vi "BlockInput8-2.vi"(3 "error in (no error)":errorcluster, 5 "BlockInput?":bool=TRUE) -> (0 "error in (no error) 2":errorcluster)   [LabVIEW 2014]
uses:
  user32.dll
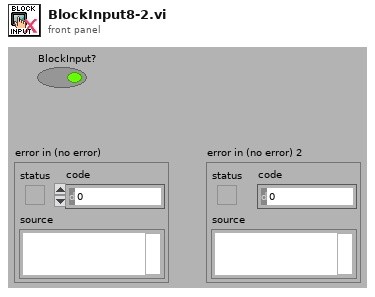
[diagram p1: front panel]
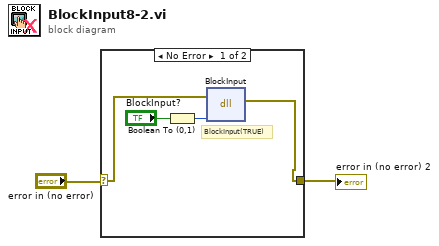
[diagram p0: block diagram]
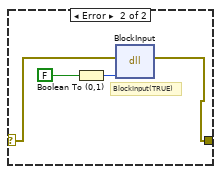
[diagram p2: hidden frame]
diagram:
  n1 = case shown="No Error" "error in (no error)" {
    selector: "error in (no error)" -> [w3 w8]
    tunnel: [w4 w7] -> w1
    frame No Error {
      # "BlockInput(TRUE)"
      n2 = Boolean To (0,1)(Boolean="BlockInput?") -> (0, 1=w6:i16)
      n3 = dll-call lib="user32.dll" fn="BlockInput"(error in=w3, "input"=w6) -> (error out=w4:errorcluster)  [unwired: 2 in, 3 out]
    }
    frame Error {
      # "BlockInput(TRUE)"
      n4 = Boolean To (0,1)(Boolean=FALSE) -> (0, 1=w10:i16)
      n5 = dll-call lib="user32.dll" fn="BlockInput"(error in=w8, "input"=w10) -> (error out=w7:errorcluster)  [unwired: 2 in, 3 out]
    }
  }
  "error in (no error) 2" <- w1
